vi "Pre Launch Init.vi"(11 "InterferometrUI in":refnum<class "InterferometerUI.lvclass">) -> (0 "error out":errorcluster, 3 "InterferometrUI out":refnum<class "InterferometerUI.lvclass">)   [LabVIEW 2023, in "InterferometrUI.lvlib" / "InterferometerUI.lvclass"]
doc: "(<B>Filename</B>: Actor Framework.lvlib:Actor.lvclass:Pre Launch Init.vi)\n\nDefines behavior that occurs after the Launch Nested Actor method is invoked but before the actor's Actor Core method begins running.\n\nBy default, this method does nothing. A descendant class may override it to define behavior."
uses:
  InterferometerUI.lvclass
  InterferometerUI.lvclass/InterferometerUI.ctl
  <vilib>/ActorFramework/Actor/Actor.lvclass
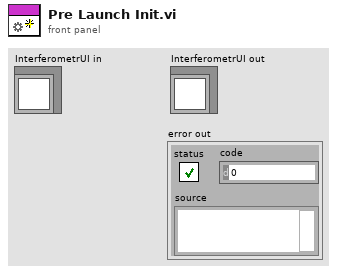
[diagram p1: front panel]
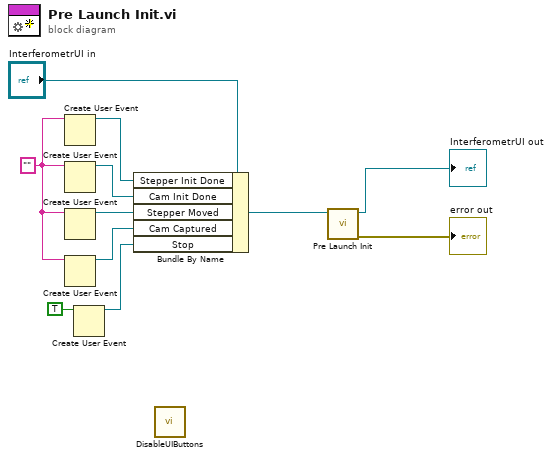
[diagram p0: block diagram]
diagram:
  w1 = ""
  n1 = Create User Event(user event datatype=w1) -> (user event=w8:refnum<user-event>)  [unwired: 1 in, 1 out]
  n2 = Create User Event(user event datatype=w1) -> (user event=w7:refnum<user-event>)  [unwired: 1 in, 1 out]
  n3 = Create User Event(user event datatype=w1) -> (user event=w6:refnum<user-event>)  [unwired: 1 in, 1 out]
  n4 = Create User Event(user event datatype=w1) -> (user event=w5:refnum<user-event>)  [unwired: 1 in, 1 out]
  n5 = Create User Event(user event datatype=TRUE) -> (user event=w4:refnum<user-event>)  [unwired: 1 in, 1 out]
  n6 = Bundle By Name(cluster="InterferometrUI in", "Stepper Init Done"=w8, "Cam Init Done"=w7, "Stepper Moved"=w6, "Cam Captured"=w5, "Stop"=w4) -> (w2:refnum<class "InterferometerUI.lvclass">)
  n7 = call "DisableUIButtons.vi"() -> ()  [unwired: 12 in]
  n8 = call-parent "Pre Launch Init.vi"("Actor in"=w2) -> ("error out"=→"error out":errorcluster, "Actor out"=→"InterferometrUI out":refnum<class "InterferometerUI.lvclass">)  [unwired: 9 in]
